vi "XY Graph to Intensity Graph (by val).vi"(6 "Y Label":string, 8 "error in (no error)":errorcluster, 9 "Y Scale":dbl[](array[numeric]), 11 "graph_utilities in":refnum<class "graph_utilities.lvclass">) -> (0 "error out":errorcluster, 3 "graph_utilities out":refnum<class "graph_utilities.lvclass">)   [LabVIEW 2019, in "graph_utilities.lvclass"]
doc: "Converts a sequence of XY Graphs to an Intensity Graph. Auomatically interpolates along X and Y."
uses:
  graph_utilities.lvclass
  <vilib>/PRIrvin/XY Utilities/xy_utilities.lvlib
panel:
  out "Z Array":dbl[][](array[numeric])
  in  "XY-data":cluster{"X-array":dbl[], "Y-array":dbl[]}[](array[cluster]) {"Y-array" format="%.2p"; "X-array" format="%.2p"}
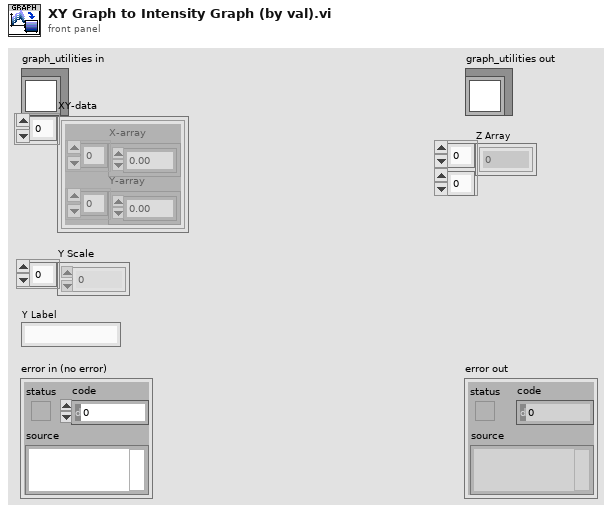
[diagram p1: front panel]
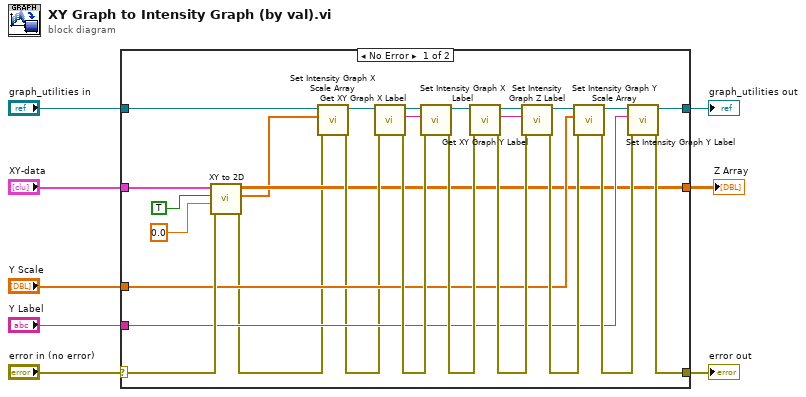
[diagram p0: block diagram]
diagram:
  n1 = case shown="No Error" "error in (no error)" {
    selector: "error in (no error)" -> [w34 w36]
    tunnel: [w20 w36] -> w7
    tunnel: [w26 w35] -> w5
    tunnel: "graph_utilities in" -> [w9 w35]
    tunnel: "Y Scale" -> [w18 _]
    tunnel: "Y Label" -> [w19 _]
    tunnel: "XY-data" -> [w13 _]
    tunnel: [w12 _] -> w1
    frame No Error {
      n2 = call <vilib>:"XY to 2D.vi"("error in (no error)"=w34, "Fake Point"=0.0, "Interpolate [T]"=TRUE, "XY-data"=w13) -> ("error out"=w10:errorcluster, "X Array"=w11:dbl[], "2D Z Array"=w12:dbl[][])  [unwired: 4 in, 1 out]
      n3 = call "Set Intensity Graph X Scale Array.vi"("error in (no error)"=w10, "X Scale"=w11, "graph_utilities in"=w9) -> ("error out"=w16:errorcluster, "graph_utilities out"=w17:refnum<class "graph_utilities.lvclass">)  [unwired: 7 in]
      n4 = call "Get XY Graph X Label.vi"("error in (no error)"=w16, "graph_utilities in"=w17) -> ("error out"=w25:errorcluster, "X Label"=w30:string, "graph_utilities out"=w31:refnum<class "graph_utilities.lvclass">)  [unwired: 7 in]
      n5 = call "Set Intensity Graph X Label.vi"("error in (no error)"=w25, "X Label"=w30, "graph_utilities in"=w31) -> ("error out"=w24:errorcluster, "graph_utilities out"=w29:refnum<class "graph_utilities.lvclass">)  [unwired: 7 in]
      n6 = call "Get XY Graph Y Label.vi"("error in (no error)"=w24, "graph_utilities in"=w29) -> ("error out"=w23:errorcluster, "Y Label"=w32:string, "graph_utilities out"=w33:refnum<class "graph_utilities.lvclass">)  [unwired: 7 in]
      n7 = call "Set Intensity Graph Z Label.vi"("error in (no error)"=w23, "Z Label"=w32, "graph_utilities in"=w33) -> ("error out"=w22:errorcluster, "graph_utilities out"=w28:refnum<class "graph_utilities.lvclass">)  [unwired: 7 in]
      n8 = call "Set Intensity Graph Y Scale Array.vi"("error in (no error)"=w22, "Y Scale"=w18, "graph_utilities in"=w28) -> ("error out"=w21:errorcluster, "graph_utilities out"=w27:refnum<class "graph_utilities.lvclass">)  [unwired: 7 in]
      n9 = call "Set Intensity Graph Y Label.vi"("error in (no error)"=w21, "Y Label"=w19, "graph_utilities in"=w27) -> ("error out"=w20:errorcluster, "graph_utilities out"=w26:refnum<class "graph_utilities.lvclass">)  [unwired: 7 in]
    }
    frame Error {
    }
  }
  "error out" <- w7
  "graph_utilities out" <- w5
  "Z Array" <- w1
